vi "Set Sampling Point.vi"(8 "error in (no error)":errorcluster, 9 "distance":u16, 10 "position":u8, 11 "Distance IR Bricklet in":refnum<class "Distance IR Bricklet.lvclass">) -> (0 "error out":errorcluster, 3 "Distance IR Bricklet out":refnum<class "Distance IR Bricklet.lvclass">)   [LabVIEW 2011, in "Tinkerforge.lvlib" / "Distance IR Bricklet.lvclass"]
doc: "This VI sets a sampling point value to a specific position of the lookup table. The lookup table is comprised of 128 equidistant analog values with corresponding distances.\n\nIf you measure a distance of 50cm at the analog value 2048, you should call this function with (64, 5000). The utilized analog to digital converter has a resolution of 12 bit. With 128 sampling points on the whole range, this means that every sampling point has a size of 32 analog values. Thus the analog value 2048 has the corresponding sampling point 64 = 2048/32.\n\nSampling points are saved on the EEPROM of the Distance-IR Bricklet and loaded again on startup."
uses:
  Distance IR Bricklet.lvclass
  Device/Device.lvclass
  IP Connection/IP Connection.lvclass
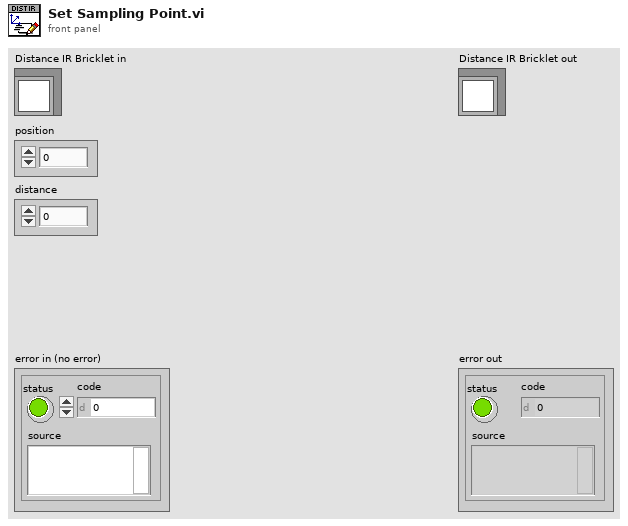
[diagram p1: front panel]
types:
  T1 = enum16{"big-endian, network order", "native, host order", "little-endian"}
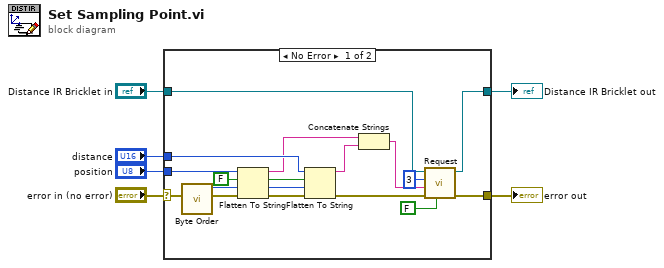
[diagram p0: block diagram]
diagram:
  n1 = case shown="No Error" "error in (no error)" {
    selector: "error in (no error)" -> [w16 w23]
    tunnel: [w17 w23] -> w5
    tunnel: [w20 w22] -> w3
    tunnel: "Distance IR Bricklet in" -> [w21 w22]
    tunnel: "position" -> [w15 _]
    tunnel: "distance" -> [w13 _]
    frame No Error {
      w12 = FALSE ("prepend array or string size? (T)")
      n2 = call "Byte Order.vi"() -> ("byte order (2:little-endian)"=w11:T1)  [unwired: 11 in]
      n3 = Flatten To String(anything=w15, prepend array or string size? (T)=w12, byte order (0:big-endian, network order)=w11, error in (no error)=w16) -> (data string=w10:string, error out=w14:errorcluster)  [unwired: 1 out]
      n4 = Flatten To String(anything=w13, prepend array or string size? (T)=w12, byte order (0:big-endian, network order)=w11, error in (no error)=w14) -> (data string=w9:string, error out=w7:errorcluster)  [unwired: 1 out]
      n5 = Concatenate Strings(w10, w9) -> (w8:string)
      n6 = call "Request.vi"("Response"=FALSE, "error in (no error)"=w7, "Data"=w8, "Function ID"=u8 3, "Device in"=w21) -> ("error out"=w17:errorcluster, "Device out"=w20:refnum<class "Distance IR Bricklet.lvclass">)  [unwired: 2 in, 3 out]
    }
    frame Error {
    }
  }
  "error out" <- w5
  "Distance IR Bricklet out" <- w3
